vi "isNull.vi"(8 "error in (no error)":errorcluster, 11 "NullCustomer in":refnum<class "NullCustomer.lvclass">) -> (0 "error out":errorcluster, 3 "NullCustomer out":refnum<class "NullCustomer.lvclass">)   [LabVIEW 2017, in "NullCustomer.lvclass"]
uses:
  NullCustomer.lvclass
  AbstractCustomer Class/AbstractCustomer.lvclass
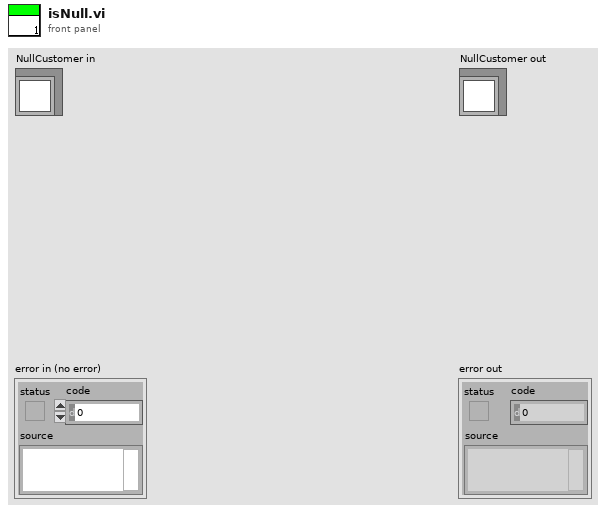
[diagram p1: front panel]
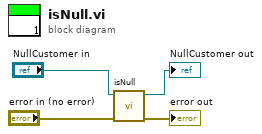
[diagram p0: block diagram]
diagram:
  n1 = call-parent "isNull.vi"("error in (no error)"="error in (no error)", "AbstractCustomer in"="NullCustomer in") -> ("error out"=→"error out":errorcluster, "AbstractCustomer out"=→"NullCustomer out":refnum<class "NullCustomer.lvclass">)  [unwired: 7 in, 1 out]
